vi "Assign GPIO.vi"(7 "SCK":refnum<class "GPIO.lvclass">, 8 "error in (no error)":errorcluster, 9 "RX":refnum<class "GPIO.lvclass">, 10 "TX":refnum<class "GPIO.lvclass">, 11 "SPI in":refnum<class "SPI.lvclass">) -> (0 "error out":errorcluster, 3 "SPI out":refnum<class "SPI.lvclass">)   [LabVIEW 2020, in "CTI.lvlib" / "SPI.lvclass"]
uses:
  SPI.lvclass
  GPIO/GPIO.lvclass
  SPI.lvclass/SPI.ctl
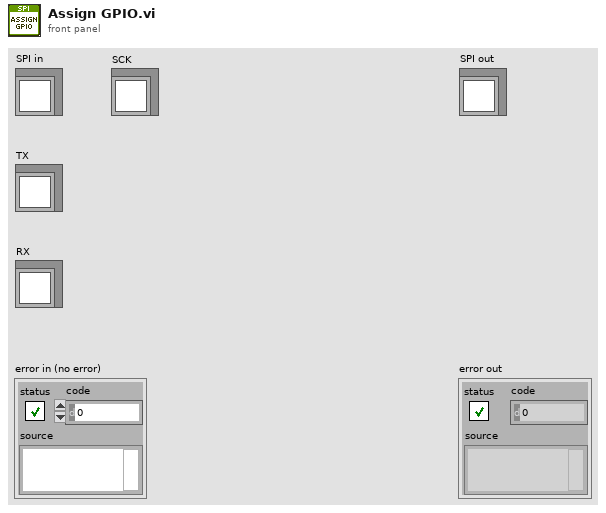
[diagram p1: front panel]
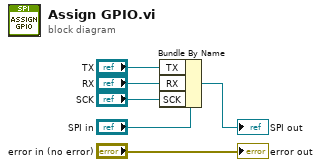
[diagram p0: block diagram]
diagram:
  n1 = Bundle By Name(cluster="SPI in", "TX"="TX", "RX"="RX", "SCK"="SCK") -> (→"SPI out":refnum<class "SPI.lvclass">)
  "error out" <- "error in (no error)"
